vi "DSF.Engine.Memory.Cache.Transfer.Initialize.vi"(8 "error in (no error)":errorcluster, 9 "Device Ref in":T1=18446744073709551615 format="%.0x", 10 "Transfer Configuration":refnum<class "DSF.Shared.Configuration.Transfer.lvclass">, 11 "Transfer Cache in":refnum<class "DSF.Engine.Memory.Cache.Transfer.lvclass">) -> (0 "error out":errorcluster, 3 "Transfer Cache out":refnum<class "DSF.Engine.Memory.Cache.Transfer.lvclass">)   [LabVIEW 2016, in "DSF.Engine.lvlib" / "DSF.Engine.Memory.Cache.Transfer.lvclass"]
uses:
  DSF.Engine.Memory.Cache.Transfer.lvclass
  Shared/Classes/Transfer/DSF.Shared.Configuration.Transfer.lvclass
  <vilib>/NI Veristand/Custom Device API/Custom Device Item Ref.ctl
  DSF.Engine.Memory.Cache.Transfer.lvclass/DSF.Engine.Memory.Cache.Transfer.ctl
  Shared/Classes/Transfer/DSF.Shared.Configuration.Transfer.lvclass/DSF.Shared.Configuration.Transfer.ctl
  Shared/Classes/Transfer/DSF.Shared.Configuration.Transfer.Required Buffer Size.vi
  DSF.Engine.Memory.Cache.Transfer.Set Buffer.vi
  DSF.Engine.Memory.Cache.Transfer.Get Configuration.vi
  DSF.Engine.Memory.Cache.Transfer.Set VS Channels Pointer.vi
  Pointer/DSF.Engine.Memory.Pointer.VS Channels.New.vi
  Shared/Classes/Transfer/DSF.Shared.Configuration.Transfer.Get Block Descriptors.vi
  Shared/Classes/Transfer/DSF.Shared.Configuration.Transfer.Get Channel Count.vi
  Shared/Classes/Transfer/DSF.Shared.Configuration.Transfer.Get Access Mode.vi
  Shared/VIs/DSF.Shared.Data Type.Sizeof.1D.vi
  Pointer/DSF.Engine.Memory.Pointer.VS Channels.Data Ref to Pointer.vi
  Shared/Classes/Transfer/DSF.Shared.Configuration.Transfer.Get Channel Descriptors.vi
  Shared/Classes/Transfer/DSF.Shared.Configuration.Transfer.Get Direction.vi
  Shared/VIs/DSF.Shared.Data Type.Sizeof.vi
  Pointer/DSF.Engine.Memory.Pointer.VS Channels.lvclass
  C:/Git/SourceTree/DSF/Source/Submodules/Memory/Source/Classes/External/Memory.Pointer.External.lvclass
  Submodules/Memory/Source/Classes/External/Memory.Pointer.External.Encapsulate.vi
  <vilib>/NI Veristand/Custom Device API/Global Data Refs.vi
  <vilib>/NI Veristand/Custom Device API/NI VeriStand - Get Channel Data Reference.vi
  Buffer/DSF.Engine.Memory.Buffer.New.vi
  <vilib>/NI Veristand/Custom Device API/Custom Device API.lvlib
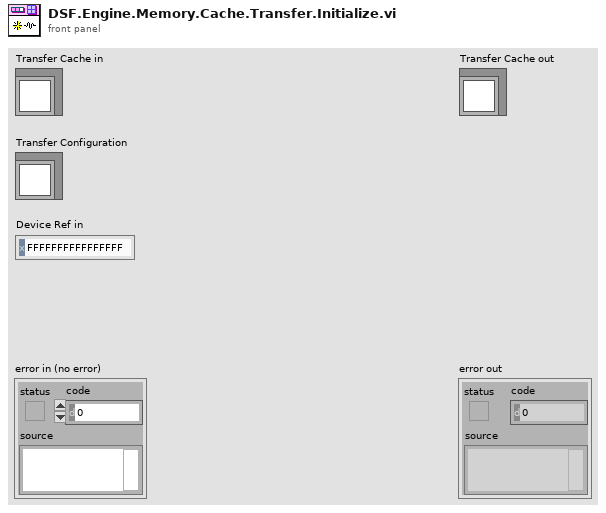
[diagram p1: front panel]
types:
  T1 = typedef "Custom Device API.lvlib/Custom Device Item Ref.ctl" = u64
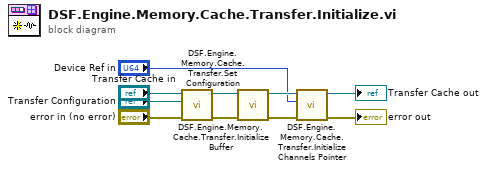
[diagram p0: block diagram]
diagram:
  n1 = call "DSF.Engine.Memory.Cache.Transfer.Set Configuration.vi"("error in (no error)"="error in (no error)", "Transfer Configuration"="Transfer Configuration", "Transfer Cache in"="Transfer Cache in") -> ("error out"=w6:errorcluster, "Transfer Cache out"=w7:refnum<class "DSF.Engine.Memory.Cache.Transfer.lvclass">)  [unwired: 7 in]
  n2 = call "DSF.Engine.Memory.Cache.Transfer.Initialize Buffer.vi"("error in (no error)"=w6, "Transfer Cache in"=w7) -> ("error out"=w4:errorcluster, "Transfer Cache out"=w5:refnum<class "DSF.Engine.Memory.Cache.Transfer.lvclass">)  [unwired: 8 in]
  n3 = call "DSF.Engine.Memory.Cache.Transfer.Initialize Channels Pointer.vi"("error in (no error)"=w4, "Device Ref in"="Device Ref in", "Transfer Cache in"=w5) -> ("error out"=→"error out":errorcluster, "Transfer Cache out"=→"Transfer Cache out":refnum<class "DSF.Engine.Memory.Cache.Transfer.lvclass">)  [unwired: 7 in]
